vi "createControls.vi"(8 "error in (no error)":errorcluster, 11 "Module in":refnum<class "Module.lvclass">) -> (0 "error out":errorcluster, 3 "Module out":refnum<class "Module.lvclass">)   [LabVIEW 2013, in "Module.lvclass"]
uses:
  Module.lvclass
  Module.lvclass/Module.ctl
  Topic/Topic.lvclass
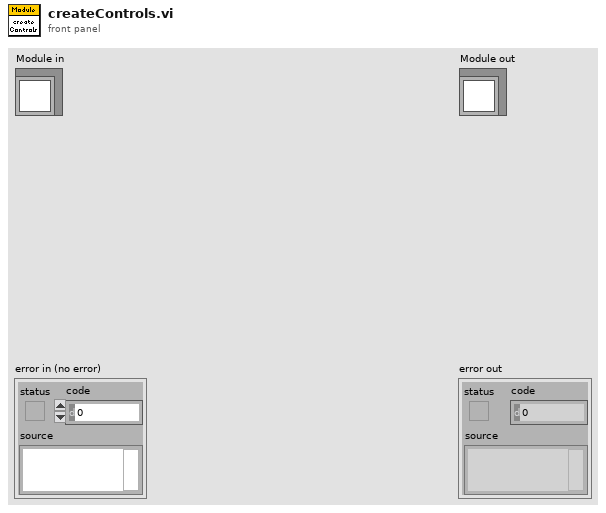
[diagram p1: front panel]
types:
  T1 = typedef "LibraryInfo.ctl" = cluster{"reference":refnum<vi>, "path":path}
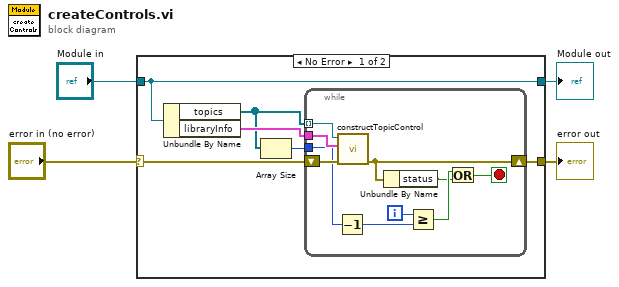
[diagram p0: block diagram]
diagram:
  n1 = case shown="No Error" "error in (no error)" {
    selector: "error in (no error)" -> [w8 w22]
    tunnel: [w7 w22] -> w3
    tunnel: [w10 w21] -> w1
    tunnel: "Module in" -> [w10 w21]
    frame No Error {
      n2 = Unbundle By Name(w10) -> ("topics"=w6:refnum<class "Topic.lvclass">[], "libraryInfo"=w9:T1)
      n3 = Array Size(array=w6) -> (size(s)=w5:i32)
      n4 = while {
        tunnel: w6 -> [w20] mode=indexing
        tunnel: w9 -> [w19]
        shift-right: [w17] -> w7
        shift-left: w8 -> [w18]
        tunnel: w5 -> [w14]
        i -> [w16]
        stop <- w11 stop-if-true
        n5 = Decrement(x=w14) -> (x-1=w15:i32)
        n6 = call "constructTopicControl.vi"("error in (no error)"=w18, "libraryInfo"=w19, "Topic in"=w20) -> ("error out"=w17:errorcluster)  [unwired: 7 in, 1 out]
        n7 = Unbundle By Name(w17) -> ("status"=w12:bool)
        n8 = Greater Or Equal?(x=w16, y=w15) -> (x >= y?=w13:bool)
        n9 = Or(x=w13, y=w12) -> (x .or. y?=w11:bool)
      }
    }
    frame Error {
    }
  }
  "error out" <- w3
  "Module out" <- w1
